vi "WaterTank(v2).vi"() -> ()   [LabVIEW 2018]
panel:
  out "Tank":dbl(slide) scale=0.0..100.0
  in  "StorValve":bool
  out "Bent1":bool
  out "Sube1":bool
  out "Tank 2":dbl(slide) scale=0.0..100.0
  out "Pump1":bool
  out "Tube6":bool
  out "Tube5":bool
  out "Tube4":bool
  out "Tube3":bool
  out "Tube2":bool
  in  "Valve1":bool
  out "Tube 1":bool
  out "Tube 14":bool
  in  "Release":bool
  out "Tube 13":bool
  in  "stop":bool
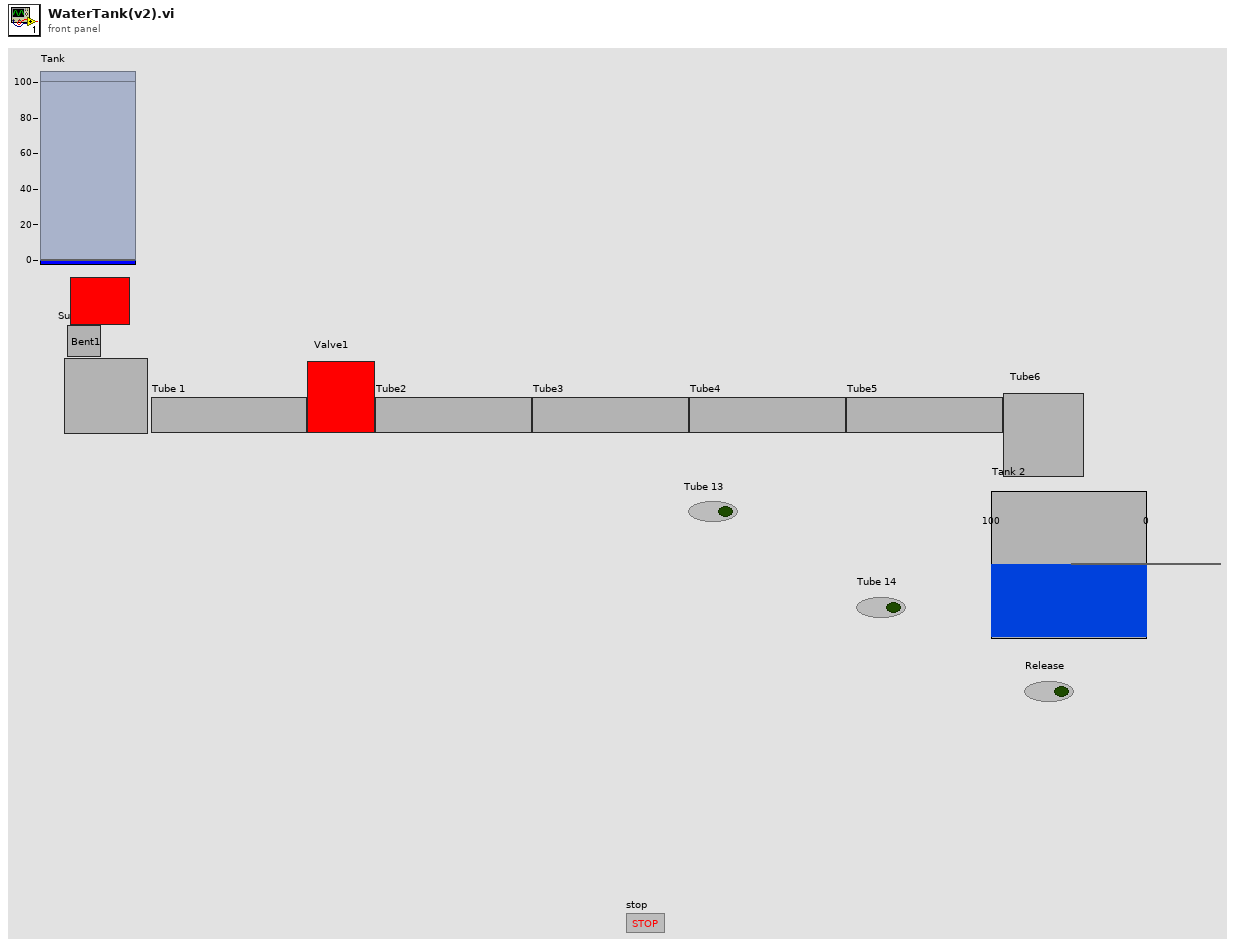
[diagram p1: front panel]
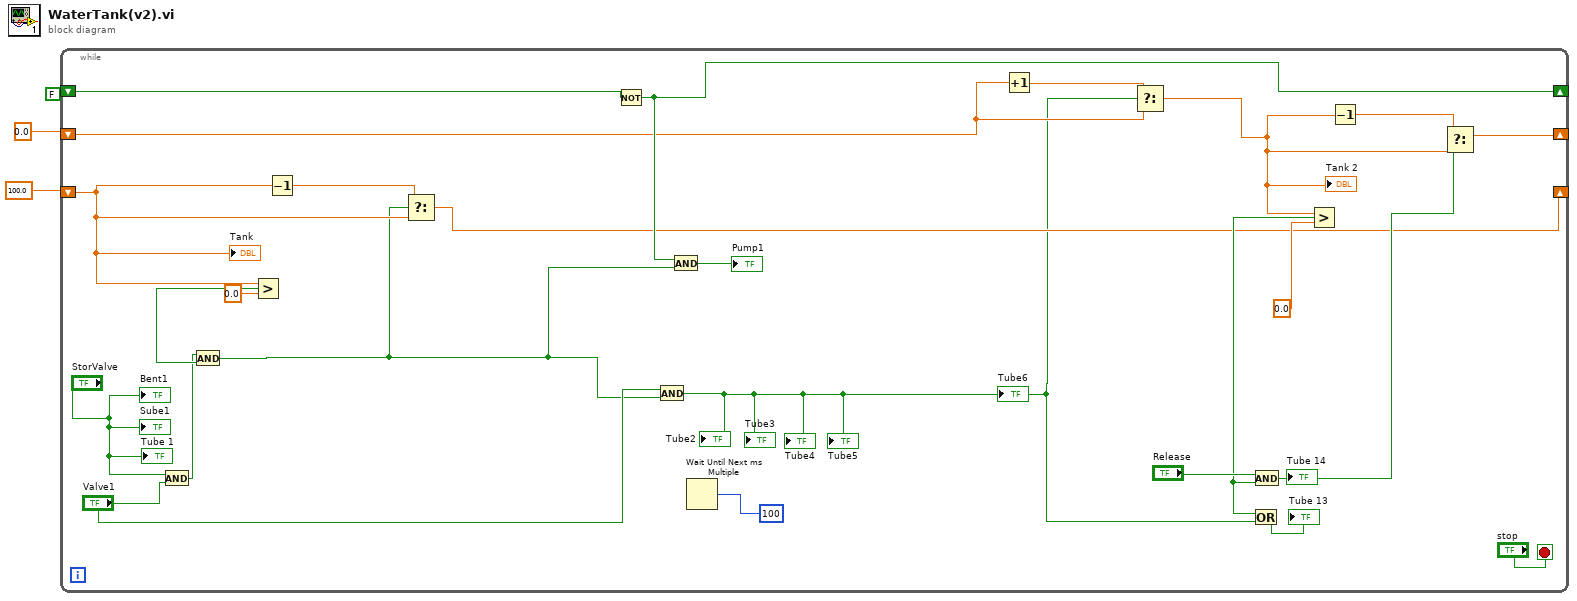
[diagram p0: block diagram]
diagram:
  (unwired) FALSE
  n1 = while {
    shift-right: [w20] -> _
    shift-left: 0.0 -> [w12]
    shift-right: [w15] -> _
    shift-left: _ -> [w14]
    shift-right: [w10] -> _
    shift-left: 100.0 -> [w9]
    stop <- "stop" stop-if-true
    n2 = And(x="StorValve", y="Valve1") -> (x .and. y?=w6:bool)
    n3 = Greater?(x=w9, y=0.0) -> (0:w7:bool)
    n4 = And(x=w6, y=w7) -> (x .and. y?=w4:bool)
    n5 = Decrement(x=w9) -> (x-1=w13:dbl)
    n6 = Select(t=w13, s=w4, f=w9) -> (s? t:f=w10:dbl)
    n7 = Not(x=w14) -> (.not. x?=w15:bool)
    n8 = And(x="Valve1", y=w4) -> (x .and. y?=w8:bool)
    "Tube2" <- w8
    "Tube3" <- w8
    "Tube4" <- w8
    "Tube5" <- w8
    "Tube6" <- w8
    n9 = And(x=w15, y=w4) -> (x .and. y?=→"Pump1":bool)
    n10 = Wait Until Next ms Multiple(millisecond multiple=100) -> ()  [unwired: 1 out]
    n11 = Increment(x=w12) -> (x+1=w27:dbl)
    n12 = Select(t=w27, s=w8, f=w12) -> (s? t:f=w17:dbl)
    "Tank 2" <- w17
    n13 = Greater?(x=w17, y=0.0) -> (0:w16:bool)
    n14 = Or(x=w16, y=w8) -> (x .or. y?=→"Tube 13":bool)
    n15 = And(x="Release", y=w16) -> (x .and. y?=w21:bool)
    "Tube 14" <- w21
    n16 = Decrement(x=w17) -> (x-1=w23:dbl)
    n17 = Select(t=w23, s=w21, f=w17) -> (s? t:f=w20:dbl)
    "Tube 1" <- "StorValve"
    "Bent1" <- "StorValve"
    "Sube1" <- "StorValve"
    "Tank" <- w9
  }
